vi "Change Module Info.vi"() -> ()   [LabVIEW 2015]
panel:
  in  "Acquisition Info":T1={"Module"="COM2", "Channels"=["FCXF-X-03-S07", "FCXF-X-03-T07", "FCXF-X-03-S08", "FCXF-X-03-T08", "FCXF-X-03-S09", "FCXF-X-03-T09", "FCXF-X-03-S10", "FCXF-X-03-T10", "FCXF-X-01-D01", "FCXF-X-01-T01", "FCXF-X-05-D01", "FCXF-X-05-T01"], "Sampling Period(S)"=600.0, "Sampling Period(Scan)"=30000, "Sampling Frequency"=30000.0} caption="采集信息" {"Sampling Frequency" format="%#_6e"}
  out "Channel Info Array":T2(array[cluster]) caption="通道信息数组"
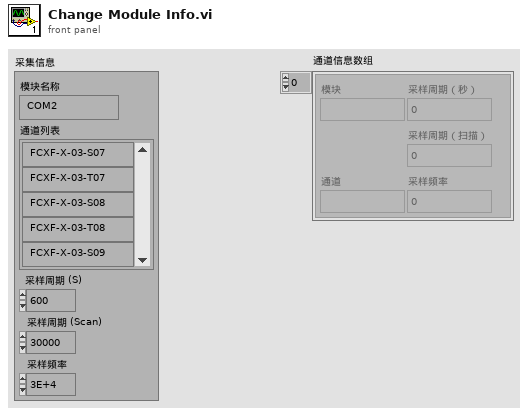
[diagram p1: front panel]
types:
  T1 = cluster{"Module":string, "Channels":string[], "Sampling Period(S)":dbl, "Sampling Period(Scan)":i64, "Sampling Frequency":dbl}
  T2 = cluster{"Module":string, "Sampling Period(S)":dbl, "Sampling Period(Scan)":i64, "Sampling Frequency":i64, "Channel":string}[]
  T3 = cluster{"Module":string, "Sampling Period(S)":dbl, "Sampling Period(Scan)":i64, "Sampling Frequency":i64, "Channel":string}
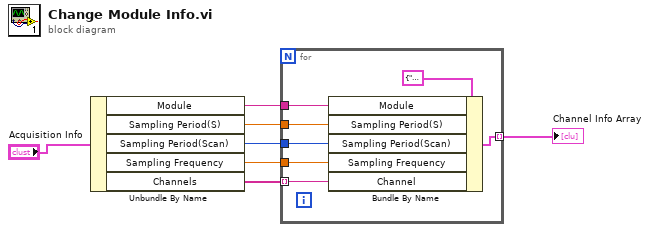
[diagram p0: block diagram]
diagram:
  n1 = Unbundle By Name("Acquisition Info") -> ("Module"=w7:string, "Sampling Period(S)"=w6:dbl, "Sampling Period(Scan)"=w5:i64, "Sampling Frequency"=w4:dbl, "Channels"=w3:string[])
  n2 = for {
    tunnel: w7 -> [w13]
    tunnel: w6 -> [w12]
    tunnel: w5 -> [w11]
    tunnel: w4 -> [w10]
    tunnel: w3 -> [w9] mode=indexing
    tunnel: [w8] -> w2 mode=indexing
    n3 = Bundle By Name(cluster=T3 {"Module"="", "Sampling Period(S)"=0.0, "Sampling Period(Scan)"=0, "Sampling Frequency"=0, "Channel"=""} ("Acquisition Info"), "Module"=w13, "Sampling Period(S)"=w12, "Sampling Period(Scan)"=w11, "Sampling Frequency"=w10, "Channel"=w9) -> (w8:T3)
  }
  "Channel Info Array" <- w2
